vi "Boolean Logic - Logic Gates.vi"() -> ()   [LabVIEW 2016]
panel:
  out "Boolean 20":bool
  in  "Boolean 19":bool
  out "Boolean 18":bool
  in  "Boolean 17":bool
  in  "Boolean 16":bool
  out "Boolean 15":bool
  in  "Boolean 14":bool
  in  "Boolean 13":bool
  out "Boolean 12":bool
  in  "Boolean 11":bool
  in  "Boolean 10":bool
  out "Boolean 9":bool
  in  "Boolean 8":bool
  in  "Boolean 7":bool
  out "Boolean 6":bool
  in  "Boolean 5":bool
  in  "Boolean 4":bool
  out "Boolean 3":bool
  in  "Boolean 2":bool
  in  "Boolean":bool
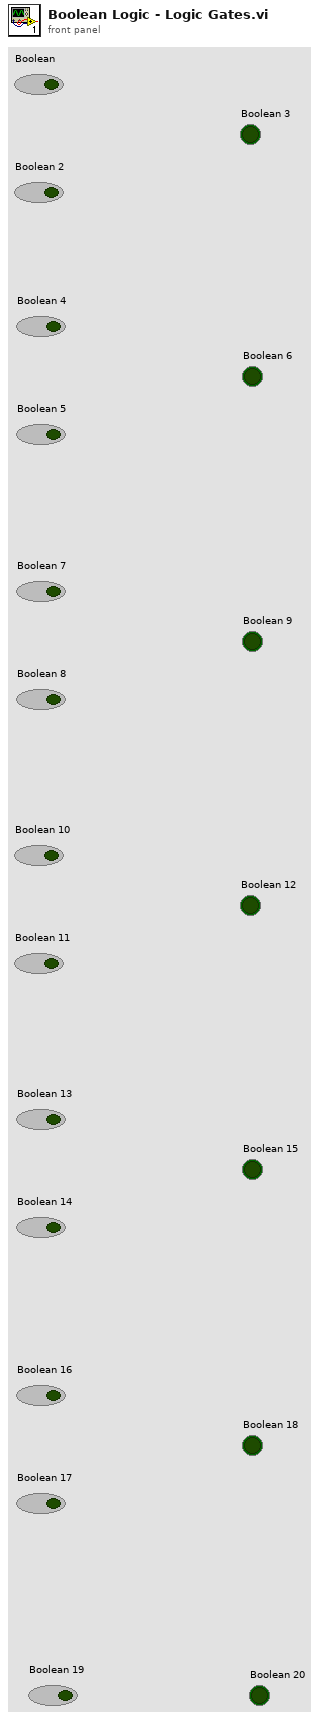
[diagram p1: front panel]
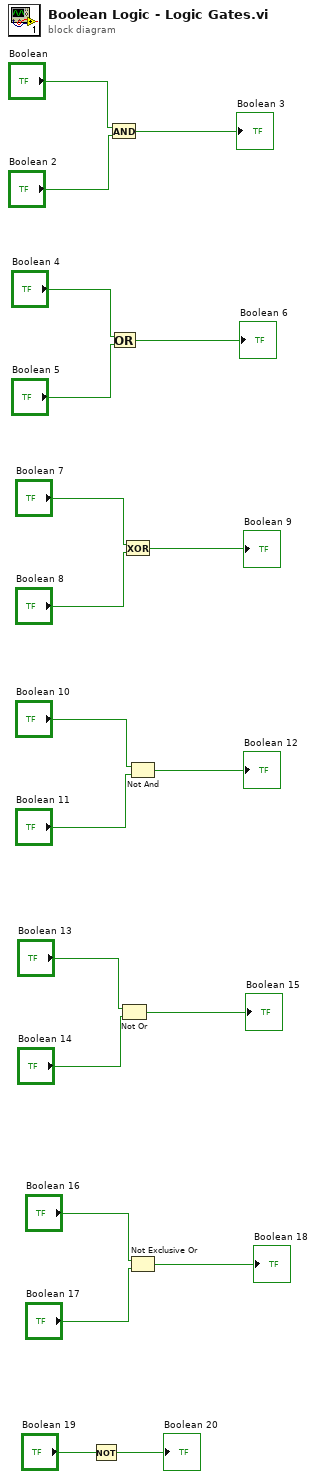
[diagram p0: block diagram]
diagram:
  n1 = Not(x="Boolean 19") -> (.not. x?=→"Boolean 20":bool)
  n2 = And(x="Boolean", y="Boolean 2") -> (x .and. y?=→"Boolean 3":bool)
  n3 = Or(x="Boolean 4", y="Boolean 5") -> (x .or. y?=→"Boolean 6":bool)
  n4 = Not Or(1:"Boolean 14", 2:"Boolean 13") -> (0:→"Boolean 15":bool)
  n5 = Exclusive Or(1:"Boolean 8", 2:"Boolean 7") -> (0:→"Boolean 9":bool)
  n6 = Not And(1:"Boolean 11", 2:"Boolean 10") -> (0:→"Boolean 12":bool)
  n7 = Not Exclusive Or(1:"Boolean 17", 2:"Boolean 16") -> (0:→"Boolean 18":bool)
